vi "DAQmx_voltage_output_autorange.vi"(0 "DAQ task Voltage Output in":refnum<k21>, 1 "Bipolar":bool, 5 "Voltage Output, V":dbl, 11 "error in (no error)":errorcluster) -> (4 "DAQ task Voltage Output out":refnum<k21>, 12 "AO.Min":dbl, 14 "AO.Max":dbl, 15 "error out":errorcluster)   [LabVIEW 2017]
uses:
  <vilib>/DAQmx/write.llb/DAQmx Write (Analog DBL 1Chan 1Samp).vi
  <vilib>/DAQmx/miscellaneous.llb/DAQmx Fill In Error Info.vi
  <resource>/objmgr/daqmx.rc
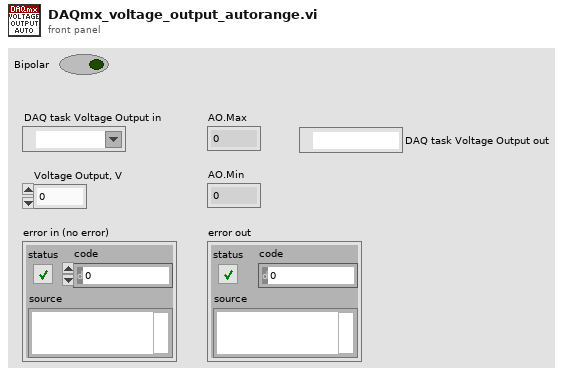
[diagram p1: front panel]
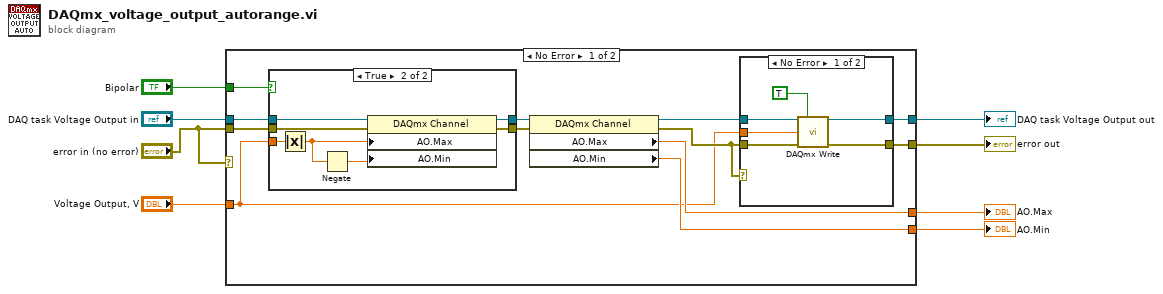
[diagram p0: block diagram]
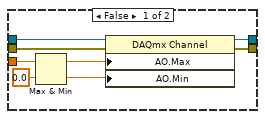
[diagram p2: hidden frame]
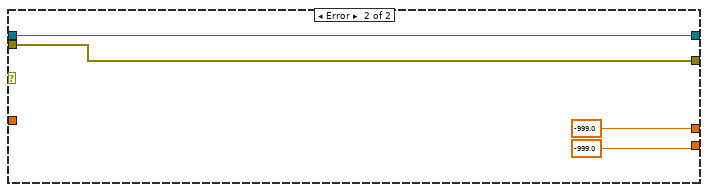
[diagram p4: hidden frame]
diagram:
  n1 = case shown="No Error" "error in (no error)" {
    tunnel: "error in (no error)" -> [w20 w46]
    tunnel: [w19 -999.0 ("AO.Min")] -> w8
    tunnel: "DAQ task Voltage Output in" -> [w18 w47]
    tunnel: [w17 -999.0 ("AO.Max")] -> w6
    tunnel: "Voltage Output, V" -> [w9 _]
    tunnel: [w13 w46] -> w4
    tunnel: [w12 w47] -> w2
    tunnel: "Bipolar" -> [w10 _]
    frame No Error {
      n2 = case shown="True" w10 {
        tunnel: w20 -> [w25 w35]
        tunnel: w18 -> [w28 w34]
        tunnel: [w26 w33] -> w15
        tunnel: [w27 w32] -> w14
        tunnel: w9 -> [w24 w30]
        frame False {
          n3 = Max & Min(x=w24, y=0.0) -> (max(x,y)=w22:dbl, min(x,y)=w21:dbl)
          n4 = property class="DAQmx Channel"(reference=w28, error in=w25, "AO.Max"=w22, "AO.Min"=w21) -> (reference out=w27:refnum<k21>, error out=w26:errorcluster)
        }
        frame True {
          n5 = Absolute Value(x=w30) -> (abs(x)=w29:dbl)
          n6 = Negate(x=w29) -> (-x=w31:dbl)
          n7 = property class="DAQmx Channel"(reference=w34, error in=w35, "AO.Max"=w29, "AO.Min"=w31) -> (reference out=w32:refnum<k21>, error out=w33:errorcluster)
        }
      }
      n8 = property class="DAQmx Channel"(reference=w14, error in=w15) -> (reference out=w16:refnum<k21>, error out=w11:errorcluster, "AO.Max"=w17:dbl, "AO.Min"=w19:dbl)
      n9 = case shown="No Error" w11 {
        tunnel: w11 -> [w41 w42]
        tunnel: w16 -> [w40 w43]
        tunnel: w9 -> [w39 _]
        tunnel: [w38 w42] -> w13
        tunnel: [w36 w43] -> w12
        frame No Error {
          n10 = call-poly <vilib>:"DAQmx Write.vi"("task/channels in"=w40, "auto start"=TRUE, "data"=w39, "error in"=w41) -> ("task out"=w36:refnum<k21>, "error out"=w38:errorcluster)  [unwired: 9 in, 1 out]
        }
        frame Error {
        }
      }
    }
    frame Error {
    }
  }
  "AO.Min" <- w8
  "AO.Max" <- w6
  "error out" <- w4
  "DAQ task Voltage Output out" <- w2
